vi "DraggingDresser.vi"() -> ()   [LabVIEW 2014]
panel:
  out "Force":dbl[](array[numeric])
  out "Angle for Minimum Force":i32 format="%.1f"
  in  "Coefficient of Kinetic Friction":dbl format="%.1f"
  out "Waveform Graph":dbl[](graph)
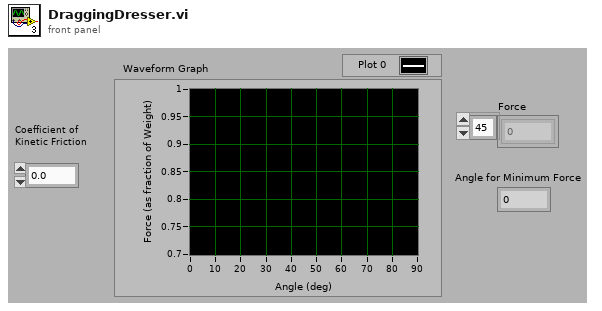
[diagram p1: front panel]
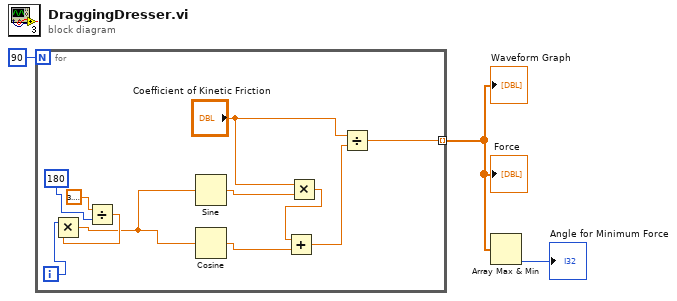
[diagram p0: block diagram]
diagram:
  n1 = for {
    N: 90 -> [_]
    tunnel: [w4] -> w2 mode=indexing
    i -> [w11]
    n2 = Divide(x=3.141592653589793, y=180) -> (x/y=w12:dbl)
    n3 = Multiply(x=w11, y=w12) -> (x*y=w10:dbl)
    n4 = Sine(x=w10) -> (sin(x)=w9:dbl)
    n5 = Cosine(x=w10) -> (cos(x)=w8:dbl)
    n6 = Multiply(x="Coefficient of Kinetic Friction", y=w9) -> (x*y=w7:dbl)
    n7 = Add(x=w7, y=w8) -> (x+y=w6:dbl)
    n8 = Divide(x="Coefficient of Kinetic Friction", y=w6) -> (x/y=w4:dbl)
  }
  "Waveform Graph" <- w2
  "Force" <- w2
  n9 = Array Max & Min(array=w2) -> (min index (indices)=→"Angle for Minimum Force":i32)  [unwired: 3 out]
